vi "ni579x Create.vi"   [LabVIEW 2014, in "ni579x Synchronization v2 FPGA.lvlib"]
uses:
  <instrlib>/ni579x/Synchronization/v2/FPGA/ni579x Synchronization v2 FPGA.lvlib
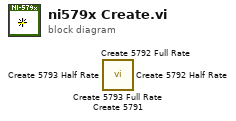
[diagram p0: block diagram]
diagram:
  n1 = call <instrlib>:"Create 5793 Full Rate.vi"() -> ()  [unwired: 15 in, 1 out]
  n2 = call <instrlib>:"Create 5792 Full Rate.vi"() -> ()  [unwired: 15 in, 1 out]
  n3 = call <instrlib>:"Create 5793 Half Rate.vi"() -> ()  [unwired: 15 in, 1 out]
  n4 = call <instrlib>:"Create 5792 Half Rate.vi"() -> ()  [unwired: 15 in, 1 out]
  n5 = call <instrlib>:"Create 5791.vi"() -> ()  [unwired: 15 in, 1 out]
